vi "readStickEnc.vi"(6 "Reset Counter":bool, 7 "Reverse ENC?":bool, 8 "error in (no error)":errorcluster) -> (0 "error out":errorcluster, 2 "StickEncoder (deg)":dbl)   [LabVIEW 2019, in "SJCube_ElvisIII.lvlib"]
uses:
  SJCube_ElvisIII.lvlib
  <vilib>/myRIO/Common/Instrument Driver Framework/myRIO v1.0/Encoder/typedefs/Encoder Signal Mode.ctl
  <vilib>/myRIO/Instrument Drivers/Onboard IO/Encoder/typedefs/Encoder Reference.ctl
  <vilib>/myRIO/Common/Instrument Driver Framework/Utilities/typedefs/myRIO Generic Hardware Reference.ctl
  <vilib>/myRIO/Common/Instrument Driver Framework/Utilities/typedefs/Hardware Version Enum.ctl
  <vilib>/myRIO/Common/Instrument Driver Framework/Utilities/typedefs/myRIO v1.0 Reference.ctl
  <vilib>/myRIO/Common/Instrument Driver Framework/Utilities/typedefs/Generic FPGA Reference.ctl
  <vilib>/myRIO/Common/Instrument Driver Framework/myRIO v1.0/Encoder/typedefs/Encoder Channels Enum.ctl
  <vilib>/myRIO/Common/Instrument Driver Framework/myRIO v1.0/Encoder/typedefs/Encoder Configuration v1.0.ctl
  <vilib>/userDefined/High Color/nirio_resource_hc.ctl
  <vilib>/myRIO/Common/Instrument Driver Framework/Utilities/vis/Is FPGA Ref Available.vi
  <vilib>/myRIO/Common/Instrument Driver Framework/ELVIS III v1.0/Encoder/vis/ELVIS III v1.1 Open Encoder.vi
  <vilib>/myRIO/Instrument Drivers/Onboard IO/Encoder/vis/Read.vi
  <vilib>/myRIO/Common/Instrument Driver Framework/Utilities/vis/Validate Channels.vi
  <vilib>/myRIO/Common/Instrument Driver Framework/ELVIS III v1.0/Encoder/vis/ELVIS III v1.0 Reserve Encoder.vi
  <vilib>/myRIO/Common/Instrument Driver Framework/ELVIS III v1.0/Encoder/vis/ELVIS III v1.0 Build MUX Configuration Encoder.vi
  <vilib>/myRIO/Common/Instrument Driver Framework/ELVIS III v1.0/Resource Manager/vis/ELVIS III v1.0 Reserve Channel List.vi
  <vilib>/myRIO/Common/Instrument Driver Framework/ELVIS III v1.0/Resource Manager/vis/ELVIS III v1.0 Create Configuration List.vi
  <vilib>/myRIO/Common/Instrument Driver Framework/ELVIS III v1.0/Resource Manager/vis/ELVIS III v1.0 Reserve Channel.vi
  <vilib>/myRIO/Common/Instrument Driver Framework/ELVIS III v1.0/Resource Manager/vis/ELVIS III v1.0 Unreserve Channel.vi
  <vilib>/myRIO/Common/Instrument Driver Framework/ELVIS III v1.0/Resource Manager/vis/ELVIS III v1.0 Build Mutex Name.vi
  <vilib>/Utility/VariantDataType/GetNumericInfo.vi
  <vilib>/Utility/error.llb/Error Cluster From Error Code.vi
  <vilib>/myRIO/Common/Instrument Driver Framework/ELVIS III v1.0/ELVIS III v1.1 Open.vi
  <vilib>/myRIO/Common/Instrument Driver Framework/Utilities/vis/IO Manager.vi
  <vilib>/myRIO/Common/Instrument Driver Framework/Utilities/vis/Configuration Manager.vi
  <vilib>/myRIO/Common/Instrument Driver Framework/ELVIS III v1.0/Resource Manager/vis/ELVIS III v1.0 Configure IO.vi
  <vilib>/myRIO/Common/Instrument Driver Framework/myRIO v1.0/myRIO v1.0 Close.vi
  <vilib>/myRIO/Common/Instrument Driver Framework/ELVIS III v1.0/Encoder/vis/ELVIS III v1.0 Configure Encoder.vi
  <vilib>/myRIO/Common/Instrument Driver Framework/ELVIS III v1.0/Encoder/vis/ELVIS III v1.0 Read Encoder.vi
  <vilib>/myRIO/Express VI/Onboard IO/Encoder/Encoder Express VI.xnode
  <vilib>/myRIO/Instrument Drivers/Onboard IO/Encoder/vis/myRIO Encoder Open.xnode
  <vilib>/myRIO/Common/Instrument Driver Framework/myRIO v1.0/Encoder/typedefs/Encoder Count Direction Enum.ctl
  <vilib>/myRIO/Instrument Drivers/Onboard IO/Encoder/Encoder.lvlib
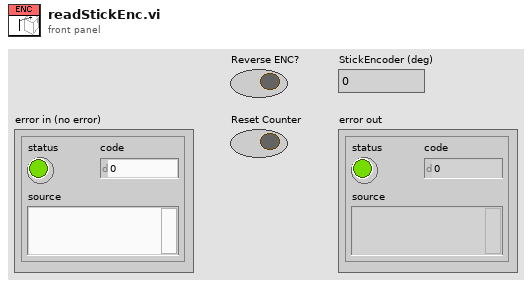
[diagram p1: front panel]
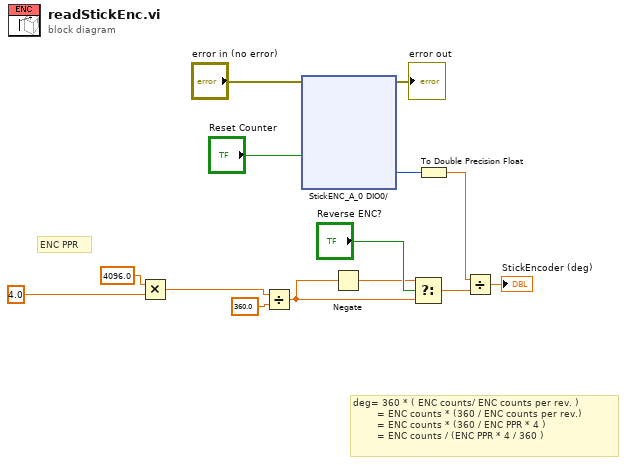
[diagram p0: block diagram]
diagram:
  # "deg= 360 * ( ENC counts/ ENC counts per rev. )\n        = ENC counts * (360 / ENC counts per rev.)\n        = ENC counts * (360 / ENC PPR * 4 )\n        = ENC counts / (ENC PPR * 4 / 360 )"
  # "ENC PPR"
  n1 = Multiply(x=4096.0 ("y"), y=4.0) -> (x*y=w3:dbl)
  n2 = Divide(x=w3, y=360.0) -> (x/y=w1:dbl)
  n3 = xnode "StickENC_A_0 DIO0/"("Reset Counter"="Reset Counter", "error in (no error)"="error in (no error)") -> ("Counter Value"=w8:i32, "error out"=→"error out":errorcluster)  [unwired: 2 out]
  n4 = Negate(x=w1) -> (-x=w6:dbl)
  n5 = Select(t=w6, s="Reverse ENC?", f=w1) -> (s? t:f=w11:dbl)
  n6 = To Double Precision Float(number=w8) -> (double precision float=w13:dbl)
  n7 = Divide(x=w13, y=w11) -> (x/y=→"StickEncoder (deg)":dbl)
